vi "GageTransfer-AdvMultiRec_Hack.vi"(0 "Handle Cluster":T1, 2 "Channels":i32=1, 3 "tail ength":u32=64, 7 "Buffer in I16":i16[](array[numeric]), 9 "Buffer in U8":u8[](array[numeric])) -> (4 "Handle Cluster out":T1, 8 "Buffer Out I16":i16[](array[numeric]), 10 "Buffer Out U8":u8[](array[numeric]), 12 "elapsed time(ms)":u32, 13 "Adj.Depth":dbl, 14 "Adj.SegmentSize":dbl, 15 "Error Code":i32)   [LabVIEW 2013]
doc: "This VI transfers the data from one channel of the CompuScope system identified by Handle Cluster, which is obtained by calling CsTool-GetSystem.vi. For accurate interpretation of the transferred data, the user should always use the returned Actual Start and Actual Length, and not the requested values. \n\nThis VI can be used for transferring data from 8, 12, 14, and 16 bit CompuScope hardware. Data are transferred from on-board CompuScope memory to PC RAM using PCI Bus Mastering at rates of up to 200 MB/s. \n\nInternally, CsTool-Transfer.vi converts the raw integer ADC code values into double variable voltage values. For more rapid data access, the user may remove the voltage conversion step. The VI will not return programmatic control to LabVIEW until all of the data have been transferred. \n\nIf the call is successful, a 1 is returned in the Error Code indicator. If the call is unsuccessful, an appropriate error code is returned. A descriptive error string may be obtained by calling CsTool-ErrorHandler.vi.\n\n\nInput Value Descriptions:\n\nChannel\nThis integer value specifies the channel from which data are to be transferred. The default value is 0 for the first channel in the CompuScope system. Channels in a LabVIEW CompuScope system begin at 0. If an invalid channel number is given, an error will be returned. Please see the CompuScope hardware manual for more information on channel enumeration.\n\nMode\nThis integer value determines the current transfer mode. Currently, the only valid value for this input is 0.\n\nSegment(1)\nThis integer value determines which Multiple Record segment is to be transferred, if the CompuScope hardware was operating in Multiple Record Mode. For Single Record Mode acquisitions, the user must always set the Record value to 1, which is the default value. If the Record value is too large, an error code will be returned. \n\nStart\nThis double variable value determines the requested starting point of the data transfer from CompuScope memory to PC RAM. Start is specified relative to the trigger address for the acquisition. A Start value of 0 will cause data transfer to begin at the trigger address. Negative Start values are used for the transfer of pre-trigger data. Positive Start values may be used to begin transfer after the trigger address. The default Start value is 0. \n\nLength\nThis double variable value specifies the amount of data, in samples, to be transferred. The default value is 4096. \n\nData in Volts\nThis array variable, of type double, is the LabVIEW buffer variable into which transferred data are returned. The size of the array will be at least Length samples. Data are returned as voltage values, whose conversion depends upon the resolution of the CompuScope system and on the current input range.\n\nActual Start\nThis double variable value returns the actual start point of the data array. The Actual Start may be lower than the requested Start value. This is because the CompuScope memory architecture may force the drivers to download data from an earlier point than the start position. For example, if Start is input to CsTool-Transfer.vi as 0, the Actual Start may return as -2, indicating that two extra samples were returned before the Start position. \n\nThe user must account for the discrepancy between the Start and the Actual Start. The user may choose to ignore samples transferred from before the Start position. Alternatively, the user may conserve these samples, accounting for the fact that the values begin at Actual Start. \n\nActual Length\nThis double variable value returns the actual amount of data transferred, which may be different from the requested Length. The difference, if any, results from CompuScope memory architecture."
panel:
  in  "Mode (0)":u32 step=1
  in  "Start (0)":dbl
  in  "Segment (1)":u32=1
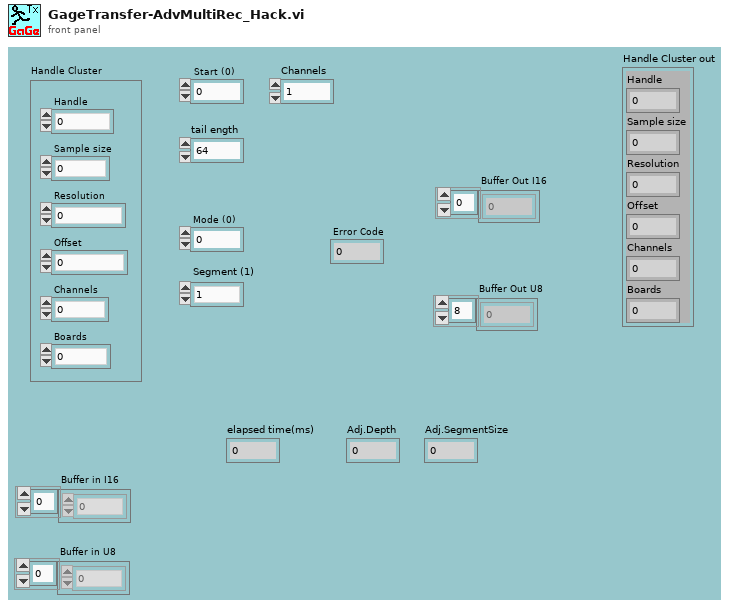
[diagram p1: front panel]
types:
  T1 = cluster{"Handle":u32, "Sample size":u32, "Resolution":i32, "Offset":i32, "Channels":u32, "Boards":u32}
  T2 = cluster{"Handle":u32, "Sample Size":u32, "Resolution":i32, "Offset":i32, "Channels":u32, "Boards":u32}
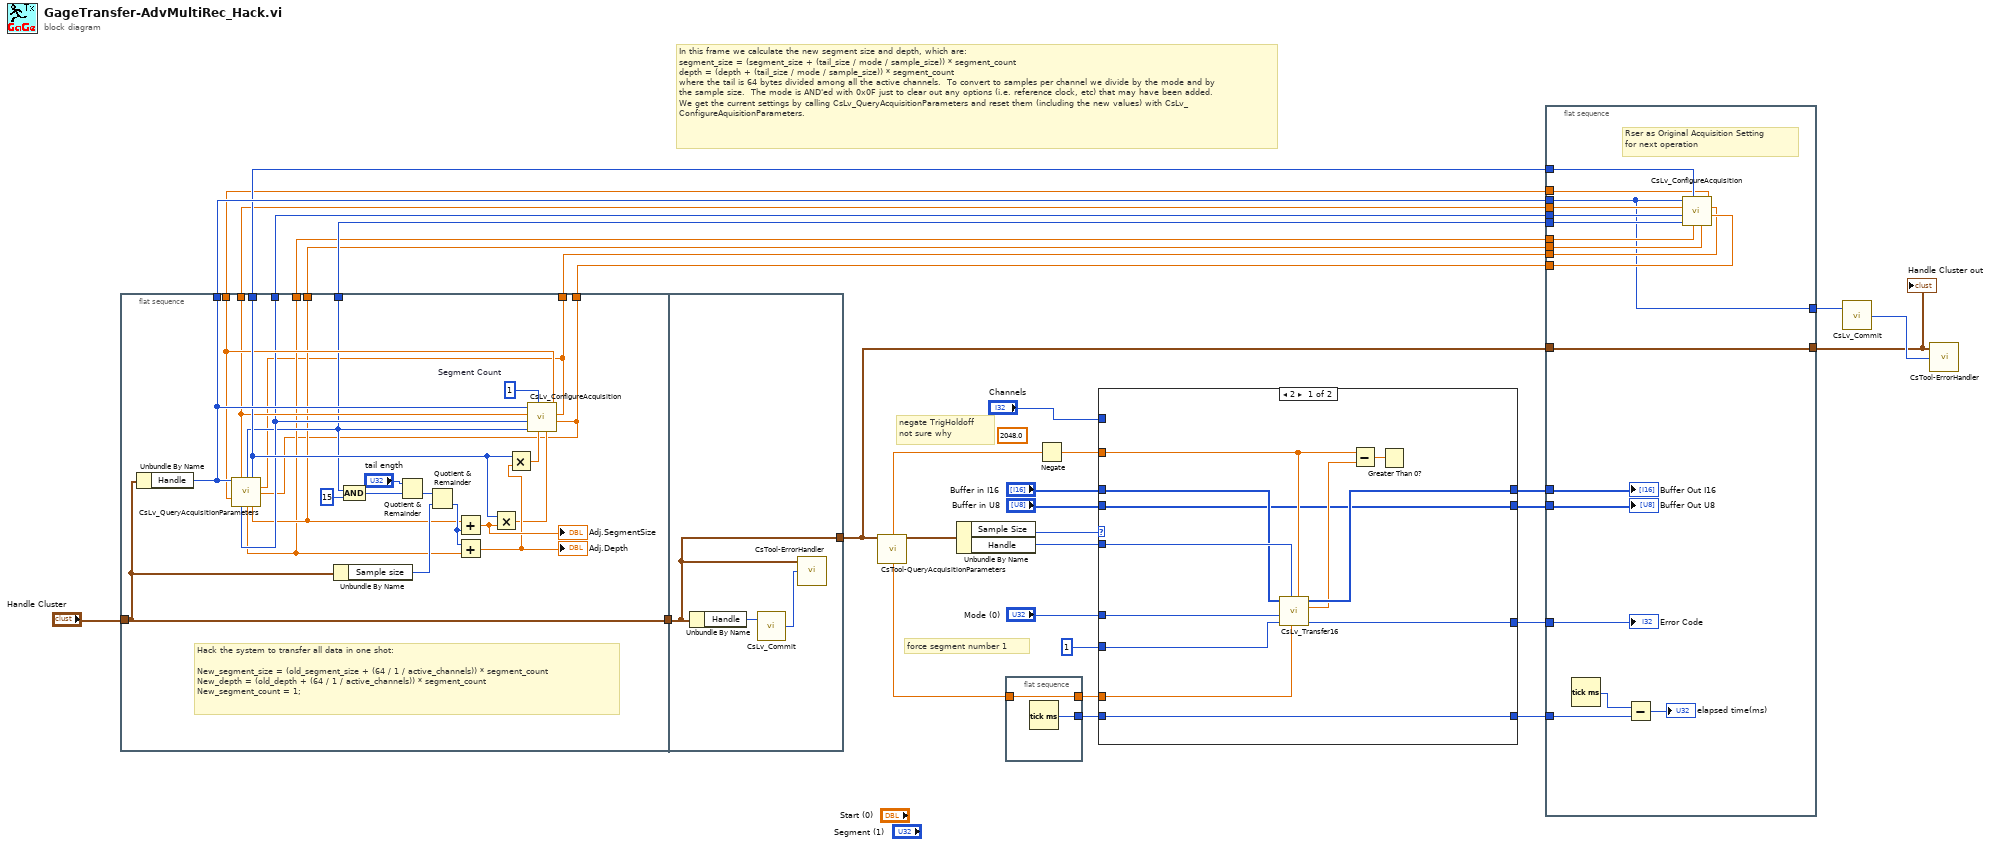
[diagram p0: block diagram]
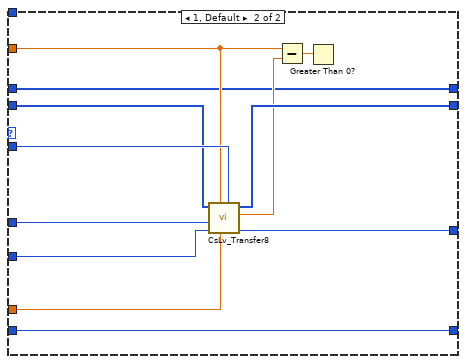
[diagram p2: hidden frame]
diagram:
  (unwired) 2048.0 ("x")
  # "force segment number 1"
  # "negate TrigHoldoff\nnot sure why"
  # "In this frame we calculate the new segment size and depth, which are:\nsegment_size = (segment_size + (tail_size / mode / sample_size)) * segment_count\ndepth = (depth + (tail_size / mode / sample_size)) * segment_count\nwhere the tail is 64 bytes divided among all the active channels.  To convert to samples per channel we divide by the mode and by the sample size.  The mode is AND'ed with 0x0F just to clear out any options (i.e. reference clock, etc) that may have been added.  We get the current settings by calling CsLv_QueryAcquisitionParameters and reset them (including the new values) with CsLv_ConfigureAquisitionParameters."
  n1 = flat-sequence {
    tunnel: "Handle Cluster" -> [w50]
    tunnel: [w50] -> w25
    tunnel: [w43] -> w20
    tunnel: [w42] -> w19
    tunnel: [w41] -> w18
    tunnel: [w40] -> w17
    tunnel: [w39] -> w16
    tunnel: [w38] -> w15
    tunnel: [w37] -> w14
    tunnel: [w36] -> w13
    tunnel: [w34] -> w12
    tunnel: [w35] -> w11
    tunnel: w25 -> [w56]
    tunnel: [w56] -> w8
    frame #0 {
      w55 = u32 1  # Segment Count
      # "Hack the system to transfer all data in one shot:\n\nNew_segment_size = (old_segment_size + (64 / 1 / active_channels)) * segment_count\nNew_depth = (old_depth + (64 / 1 / active_channels)) * segment_count\nNew_segment_count = 1;"
      n2 = Unbundle By Name(w50) -> ("Handle"=w43:u32)
      n3 = call <instrlib>:"CsLv_QueryAcquisitionParameters.vi"("Handle"=w43) -> ("Sample Rate"=w40:dbl, "Mode"=w38:u32, "Segment Count"=w42:u32, "Trigger Timeout"=w35:dbl, "Trigger Holdoff"=w34:dbl, "Trigger Delay"=w41:dbl, "Ext. Clock"=w39:u32, "Depth"=w36:dbl, "Segment Size"=w37:dbl)  [unwired: 2 in, 4 out]
      n4 = Unbundle By Name(w50) -> ("Sample size"=w49:u32)
      n5 = And(x=w38, y=u32 15) -> (x .and. y?=w45:u32)
      n6 = Quotient & Remainder(x="tail ength", y=w45) -> (floor(x/y)=w48:u32)  [unwired: 1 out]
      n7 = Quotient & Remainder(x=w48, y=w49) -> (floor(x/y)=w47:u32)  [unwired: 1 out]
      n8 = Add(x=w37, y=w47) -> (x+y=w53:dbl)
      "Adj.SegmentSize" <- w53
      n9 = Add(x=w47, y=w36) -> (x+y=w52:dbl)
      "Adj.Depth" <- w52
      n10 = Multiply(x=w42, y=w53) -> (x*y=w44:dbl)
      n11 = Multiply(x=w42, y=w52) -> (x*y=w51:dbl)
      n12 = call <instrlib>:"CsLv_ConfigureAcquisition.vi"("Trigger Holdoff (0)"=w34, "Trigger Timeout (10000000)"=w35, "Trigger Delay (0)"=w41, "Segment Size (8192)"=w44, "Depth (8192)"=w51, "Segment Count (1)"=w55, "Mode (2)"=w38, "External Clock (0)"=w39, "Sample Rate (100000000)"=w40, "Handle"=w43) -> ()  [unwired: 1 in, 1 out]
    }
    frame #1 {
      n13 = Unbundle By Name(w56) -> ("Handle"=w58:u32)
      n14 = call <instrlib>:"CsLv_Commit.vi"("Handle"=w58) -> ("Error Code"=w57:i32)  [unwired: 1 in]
      n15 = call <instrlib>:"CsTool-ErrorHandler.vi"("Error Code"=w57, "Handle Cluster"=w56) -> ()  [unwired: 1 in, 1 out]
    }
  }
  n16 = call <instrlib>:"CsTool-QueryAcquisitionParameters.vi"("Handle Cluster"=w8) -> ("Trigger Holdoff"=w5:dbl, "Output Handle Cluster"=w21:T2, "Segment Size"=w3:dbl)  [unwired: 4 in, 8 out]
  n17 = Unbundle By Name(w21) -> ("Sample Size"=w33:u32, "Handle"=w32:u32)
  n18 = flat-sequence {
    tunnel: [w60] -> w4
    tunnel: w3 -> [w60]
    tunnel: [w59] -> w1
    frame #0 {
      n19 = Tick Count (ms)() -> (millisecond timer value=w59:u32)
    }
  }
  n20 = Negate(x=w5) -> (-x=w22:dbl)
  n21 = case shown="2" w33 {
    tunnel: u32 1 ("Segment (1)") -> [w70 w82]
    tunnel: "Mode (0)" -> [w69 w81]
    tunnel: w22 -> [w68 w80]
    tunnel: [w72 w84] -> w30
    tunnel: w32 -> [w71 w83]
    tunnel: "Buffer in U8" -> [w63 w79]
    tunnel: "Buffer in I16" -> [w67 w75]
    tunnel: [w66 w75] -> w27
    tunnel: [w63 w78] -> w26
    tunnel: "Channels" -> [_ _]
    tunnel: w4 -> [w61 w74]
    tunnel: [w62 w73] -> w2
    tunnel: w1 -> [w62 w73]
    frame 2 {
      n22 = call <instrlib>:"CsLv_Transfer16.vi"("Start (0)"=w68, "Length (4096)"=w61, "Handle"=w71, "Segment (1)"=w70, "Mode (0)"=w69, "Buffer in I16"=w67) -> ("Error Code"=w72:i32, "Actual Start"=w64:dbl, "Buffer"=w66:i16[])  [unwired: 2 in, 1 out]
      n23 = Subtract(x=w68, y=w64) -> (x-y=w65:dbl)
      n24 = Greater Than 0?(x=w65) -> ()  [unwired: 1 out]
    }
    frame 1, Default {
      n25 = call <instrlib>:"CsLv_Transfer8.vi"("Handle"=w83, "Length (4096)"=w74, "Start (0)"=w80, "Segment (1)"=w82, "Mode (0)"=w81, "Buffer in"=w79) -> ("Error Code"=w84:i32, "Actual Start"=w76:dbl, "Buffer out"=w78:u8[])  [unwired: 2 in, 1 out]
      n26 = Subtract(x=w80, y=w76) -> (x-y=w77:dbl)
      n27 = Greater Than 0?(x=w77) -> ()  [unwired: 1 out]
    }
  }
  n28 = flat-sequence {
    tunnel: w30 -> [w101]
    tunnel: w27 -> [w100]
    tunnel: w26 -> [w99]
    tunnel: w20 -> [w89]
    tunnel: w19 -> [w98]
    tunnel: w18 -> [w97]
    tunnel: w17 -> [w96]
    tunnel: w16 -> [w95]
    tunnel: w15 -> [w94]
    tunnel: w14 -> [w93]
    tunnel: w13 -> [w92]
    tunnel: w12 -> [w91]
    tunnel: w11 -> [w90]
    tunnel: [w89] -> w9
    tunnel: w8 -> [w88]
    tunnel: [w88] -> w7
    tunnel: w2 -> [w87]
    frame #0 {
      # "Rser as Original Acquisition Setting\nfor next operation"
      n29 = Tick Count (ms)() -> (millisecond timer value=w86:u32)
      n30 = Subtract(x=w86, y=w87) -> (x-y=→"elapsed time(ms)":u32)
      n31 = call <instrlib>:"CsLv_ConfigureAcquisition.vi"("Trigger Holdoff (0)"=w91, "Trigger Timeout (10000000)"=w90, "Trigger Delay (0)"=w97, "Segment Size (8192)"=w93, "Depth (8192)"=w92, "Segment Count (1)"=w98, "Mode (2)"=w94, "External Clock (0)"=w95, "Sample Rate (100000000)"=w96, "Handle"=w89) -> ()  [unwired: 1 in, 1 out]
      "Buffer Out U8" <- w99
      "Error Code" <- w101
      "Buffer Out I16" <- w100
    }
  }
  n32 = call <instrlib>:"CsLv_Commit.vi"("Handle"=w9) -> ("Error Code"=w10:i32)  [unwired: 1 in]
  n33 = call <instrlib>:"CsTool-ErrorHandler.vi"("Error Code"=w10, "Handle Cluster"=w7) -> ()  [unwired: 1 in, 1 out]
  "Handle Cluster out" <- w7
